vi "WPI_GyroXRS450_SPI_Open.vi"(6 "Calibrated Center Offset":dbl, 7 "Calibration Time (s)":dbl=2.0, 8 "error in":errorcluster, 9 "Calibrate On Open":bool=TRUE, 10 "Sample Rate (Hz)":dbl=2000.0, 11 "SPI Bus":T3) -> (0 "error out":errorcluster, 2 "Calibrated Center Offset Out":dbl, 3 "GyroDevRef":T1={"DevStatus"={"status"=FALSE, "code"=0, "source"=""}, "Analog Channel"=enum."AI 0", "Gain (VoltsPerDegree/Second)"=0.0, "Gyro Type"=enum."Analog", "Handle"=0, "SPI Bus"=enum."Invalid", "Device Found"=FALSE, "Sample Rate"=1.0, "Calibrate On Open"=FALSE, "Offset"=0.0} {"Sample Rate" min=0.25 max=100.0 step=0.25})   [LabVIEW 2017]
doc: "Opens a reference to the gyroscope you specify. You must open a reference before using any other VIs on this palette.\n\nThis software is licensed. Open the labview\\readme\\WPI Robotics Library Open Source License.txt file for more information."
uses:
  <vilib>/Rock Robotics/SystemInterfaces/spilib/spi_bus.ctl
  <vilib>/Rock Robotics/WPI/Gyro/WPI_GyroDevRef.ctl
  <vilib>/Rock Robotics/SystemInterfaces/AI/FPGA_AIChannel.ctl
  <vilib>/Rock Robotics/WPI/SPI/WPI_SPIMode.ctl
  <vilib>/Rock Robotics/WPI/Gyro/ADXRS453/WPI_Gyro_ADXRS453_Commands.ctl
  <vilib>/Rock Robotics/WPI/Gyro/ADXRS453/WPI_Gyro_ADXRS453_Registers.ctl
  <vilib>/Rock Robotics/SystemInterfaces/NetworkCommunication/NetComm_UsageReport_ResourceType.ctl
  <vilib>/Analysis/baseanly.llb/Mean (DBL).vi
  <vilib>/Analysis/NI_AALBase.lvlib
panel:
  # "Analog"
  # "XRS"
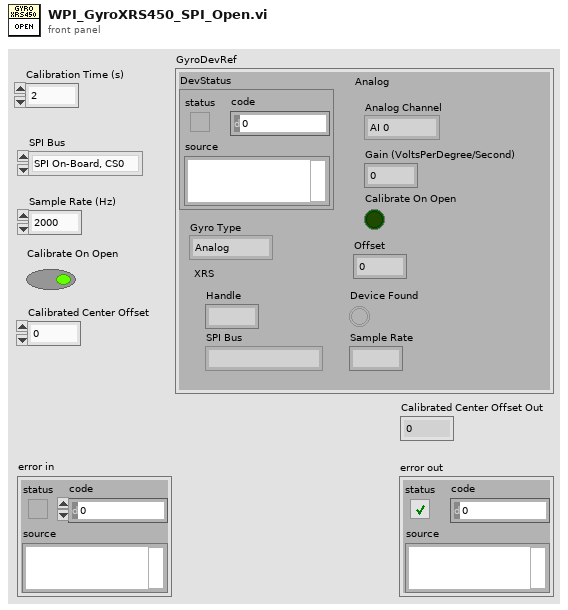
[diagram p1: front panel]
types:
  T1 = typedef "WPI_GyroDevRef.ctl" = cluster{"DevStatus":errorcluster, "Analog Channel":T2, "Gain (VoltsPerDegree/Second)":dbl, "Gyro Type":enum16{"Analog", "XRS450"}, "Handle":i32, "SPI Bus":T3, "Device Found":bool, "Sample Rate":dbl, "Calibrate On Open":bool, "Offset":dbl}
  T2 = typedef "FPGA_AIChannel.ctl" = enum8{"AI 0", "AI 1", "AI 2", "AI 3", "AI MXP 0", "AI MXP 1", "AI MXP 2", "AI MXP 3", "Invalid"}
  T3 = typedef "spi_bus.ctl" = enum16{"SPI On-Board, CS0", "SPI On-Board, CS1", "SPI On-Board, CS2", "SPI On-Board, CS3", "SPI MXP", "Invalid"}
  T4 = typedef "WPI_Gyro_ADXRS453_Commands.ctl" = u8
  T5 = typedef "WPI_SPIMode.ctl" = enum16{"Mode 0 (Clk Idle Low,Sample on Leading)", "Mode 1 (Clk Idle Low,Sample on Trailing)", "Mode 2 (Clk Idle High,Sample on Leading)", "Mode 3 (Clk Idle High,Sample on Trailing)"}
  T6 = typedef "NetComm_UsageReport_ResourceType.ctl" = enum8{"Controller", "Module", "Language", "CANPlugin", "Accelerometer", "ADXL345", "AnalogChannel", "AnalogTrigger", "AnalogTriggerOutput", "CANJaguar", "Compressor", "Counter", "Dashboard", "DigitalInput", "DigitalOutput", "DriverStationCIO", "DriverStationEIO", "DriverStationLCD", "Encoder", "GearTooth", "Gyro", "I2C", "Framework", "Jaguar", "Joystick", "Kinect", "KinectStick", "PIDController", "Preferences", "PWM", "Relay", "RobotDrive", "SerialPort", "Servo", "Solenoid", "SPI", "Task", "Ultrasonic", "Victor", "Button", "Command", "AxisCamera", "PCVideoServer", "SmartDashboard", "Talon", "HiTechnicColorSensor", "HiTechnicAccel", "HiTechnicCompass", "SRF08", "AnalogOutput", "Victor SP", "Talon SRX", "CAN Talon SRX", "ADXL362 Accel", "ADXRS450 Gyro", "Rev SPARK", "Mindsensors SD540", "Digital Filter", "ADIS16448", "PDP", "PCM", "PigeonIMU", "Nidec Brushless", "CTRE CANifier", "CTRE Future 0", "CTRE Future 1", "CTRE Future 2", "CTRE Future 3", "CTRE Future 4", "CTRE Future 5", "CTRE Future 6"}
  T7 = typedef "WPI_Gyro_ADXRS453_Registers.ctl" = u16
  T8 = typedef "WPI_SPIDevRef.ctl" = cluster{"DevStatus":errorcluster, "Handle":i32, "SPI Bus":T3}
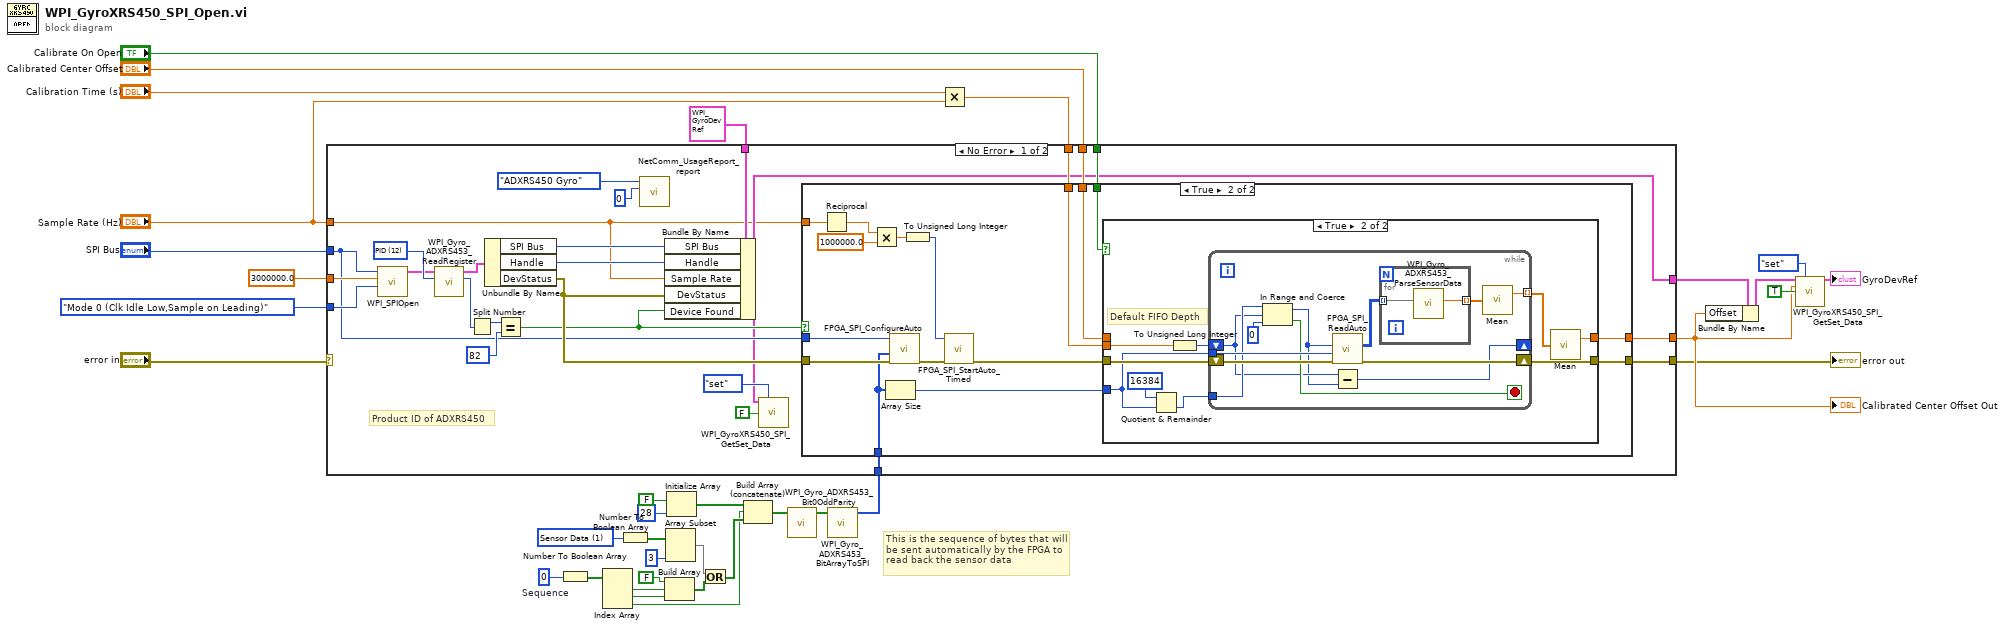
[diagram p0: block diagram]
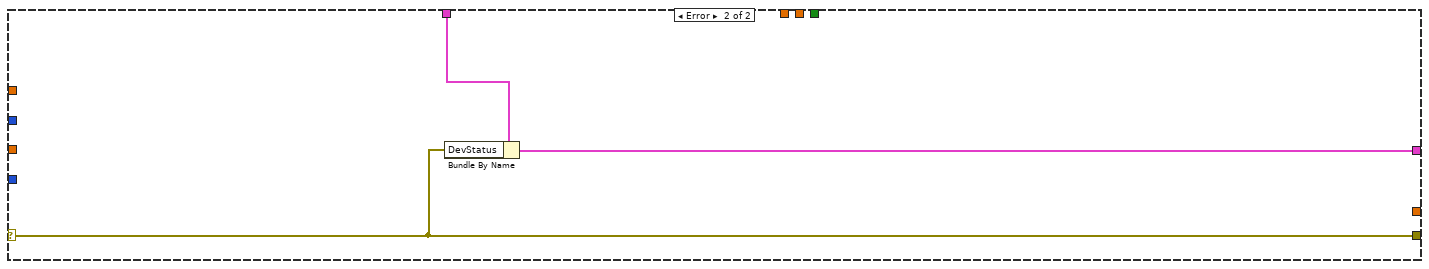
[diagram p4: hidden frame]
diagram:
  w23 = u8 0  # Sequence
  w24 = T4 1 items=["Read"=4, "Write"=2, "Sensor Data"=1]
  # "This is the sequence of bytes that will be sent automatically by the FPGA to read back the sensor data"
  n1 = Number To Boolean Array(number=w23) -> (Boolean array=w22:bool[])
  n2 = Index Array(array=w22) -> (element #1=w21:bool, element #2=w20:bool, element #3=w15:bool)  [unwired: 3 in]
  n3 = Number To Boolean Array(number=w24) -> (Boolean array=w25:bool[])
  n4 = Build Array(FALSE, w21, w20) -> (w18:bool[])
  n5 = Array Subset(array=w25, length=3) -> (w17:bool[])  [unwired: 1 in]
  n6 = Initialize Array(FALSE, 28 ("dimension size")) -> (w30:bool[])
  n7 = Or(x=w17, y=w18) -> (x .or. y?=w16:bool[])
  n8 = Build Array (concatenate)(w30, w15, w16) -> (w29:bool[])
  n9 = call <vilib>:"WPI_Gyro_ADXRS453_Bit0OddParity.vi"("Array in"=w29) -> ("Array out"=w31:bool[])  [unwired: 10 in]
  n10 = call <vilib>:"WPI_Gyro_ADXRS453_BitArrayToSPI.vi"("32-bit Array in"=w31) -> ("SPI Byte Array (MSB first)"=w8:u8[])  [unwired: 10 in]
  n11 = Multiply(x="Calibration Time (s)", y="Sample Rate (Hz)") -> (x*y=w10:dbl)
  n12 = case shown="No Error" "error in" {
    selector: "error in" -> [_ w104]
    tunnel: "SPI Bus" -> [w47 _]
    tunnel: 3000000.0 ("Clock Rate (Hz)") -> [w61 _]
    tunnel: WPI_SPIMode."Mode 0 (Clk Idle Low,Sample on Leading)" ("Mode (3)") -> [w60 _]
    tunnel: T1 {"DevStatus"={"status"=FALSE, "code"=0, "source"=""}, "Analog Channel"=enum."AI 1", "Gain (VoltsPerDegree/Second)"=0.0, "Gyro Type"=enum."XRS450", "Handle"=0, "SPI Bus"=enum."Invalid", "Device Found"=FALSE, "Sample Rate"=1.0, "Calibrate On Open"=FALSE, "Offset"=0.0} ("GyroDeviceRef") -> [w59 w106]
    tunnel: [w37 w105] -> w14
    tunnel: "Sample Rate (Hz)" -> [w36 _]
    tunnel: w8 -> [w43 _]
    tunnel: "Calibrate On Open" -> [w46 _]
    tunnel: w10 -> [w45 _]
    tunnel: "Calibrated Center Offset" -> [w44 _]
    tunnel: [w42 _] -> w4
    tunnel: [w41 w104] -> w3
    frame No Error {
      w55 = T7 12 items=["Rate"=0, "Tem"=2, "LoCST"=4, "HiCST"=6, "Quad"=8, "Fault"=10, "PID"=12, "SN High"=14, "SN Low"=16]
      # "Product ID of ADXRS450"
      n13 = call <vilib>:"WPI_SPIOpen.vi"("Mode (3)"=w60, "Clock Rate (Hz)"=w61, "SPI Bus"=w47) -> ("SPIDevRef"=w51:T8)  [unwired: 7 in, 1 out]
      n14 = call <vilib>:"WPI_Gyro_ADXRS453_ReadRegister.vi"("ADXRS453 Register"=w55, "SPIDevRef in"=w51) -> ("Register Value"=w54:u16, "SPIDevRef out"=w50:T8)  [unwired: 7 in, 1 out]
      n15 = Split Number(x=w54) -> (hi(x)=w53:u8)  [unwired: 1 out]
      n16 = Unbundle By Name(w50) -> ("SPI Bus"=w58:T3, "Handle"=w57:i32, "DevStatus"=w56:errorcluster)
      n17 = Equal?(x=w53, y=u8 82) -> (x = y?=w40:bool)
      n18 = call <vilib>:"NetComm_UsageReport_report.vi"("Instance Number"=u8 0, "Resource Type"=NetComm_UsageReport_ResourceType."ADXRS450 Gyro") -> ()  [unwired: 10 in]
      n19 = Bundle By Name(cluster=w59, "SPI Bus"=w58, "Handle"=w57, "Sample Rate"=w36, "DevStatus"=w56, "Device Found"=w40) -> (w37:T1)
      n20 = call <vilib>:"WPI_GyroXRS450_SPI_GetSet_Data.vi"("GyroDeviceRef"=w37, "Operation"=enum16{"set", "get"}."set", "Calibrated"=FALSE) -> ()  [unwired: 8 in, 5 out]
      n21 = case shown="True" w40 {
        tunnel: w56 -> [w62 w78]
        tunnel: w47 -> [_ w77]
        tunnel: w36 -> [_ w72]
        tunnel: w46 -> [_ w70]
        tunnel: w45 -> [_ w69]
        tunnel: w44 -> [_ w68]
        tunnel: w43 -> [_ w66]
        tunnel: [_ w65] -> w42
        tunnel: [w62 w64] -> w41
        frame False {
        }
        frame True {
          n22 = Reciprocal(x=w72) -> (1/x=w63:dbl)
          n23 = Multiply(x=w63, y=1000000.0 ("x")) -> (x*y=w75:dbl)
          n24 = Array Size(array=w66) -> (size(s)=w71:i32)
          n25 = call <vilib>:"FPGA_SPI_ConfigureAuto.vi"("error in"=w78, "SPI Auto TX Byte Array"=w66, "SPI Bus"=w77) -> ("error out"=w74:errorcluster)  [unwired: 8 in]
          n26 = To Unsigned Long Integer(number=w75) -> (unsigned 32bit integer=w76:u32)
          n27 = call <vilib>:"FPGA_SPI_StartAuto_Timed.vi"("error in (no error)"=w74, "Sample Period (us)"=w76) -> ("error out"=w67:errorcluster)  [unwired: 9 in]
          n28 = case shown="True" w70 {
            tunnel: w69 -> [_ w89]
            tunnel: w68 -> [w80 _]
            tunnel: [w80 w82] -> w65
            tunnel: w67 -> [w79 w88]
            tunnel: w71 -> [_ w83]
            tunnel: [w79 w86] -> w64
            frame False {
            }
            frame True {
              # "Default FIFO Depth"
              n29 = Quotient & Remainder(x=u32 16384 ("unsigned 32bit integer"), y=w83) -> (floor(x/y)=w81:u32)  [unwired: 1 out]
              n30 = To Unsigned Long Integer(number=w89) -> (unsigned 32bit integer=w87:u32)
              n31 = while {
                tunnel: [w97] -> w85 mode=indexing
                tunnel: w83 -> [w96]
                shift-right: [w98] -> w86
                shift-left: w88 -> [w100]
                tunnel: w81 -> [w95]
                shift-right: [w90] -> _
                shift-left: w87 -> [w92]
                stop <- w93 stop-if-true
                n32 = In Range and Coerce(upper limit=w95, x=w92, lower limit=u32 0) -> (coerced(x)=w91:u32, In Range?=w93:bool)
                n33 = call <vilib>:"FPGA_SPI_ReadAuto.vi"("error in (no error)"=w100, "Bytes per Sample"=w96, "Samples to Read"=w91) -> ("error out"=w98:errorcluster, "Data"=w99:u8[][])  [unwired: 7 in]
                n34 = Subtract(x=w92, y=w91) -> (x-y=w90:u32)
                n35 = for {
                  tunnel: w99 -> [w103] mode=indexing
                  tunnel: [w102] -> w101 mode=indexing
                  # "Offset Calibration"
                  n36 = call <vilib>:"WPI_Gyro_ADXRS453_ParseSensorData.vi"("Data"=w103) -> ("Angular Rate (deg/sec)"=w102:dbl)  [unwired: 8 in, 2 out]
                }
                n37 = call-poly <vilib>:"Mean.vi"("X"=w101) -> ("mean"=w97:dbl)  [unwired: 1 out]
              }
              n38 = call-poly <vilib>:"Mean.vi"("X"=w85) -> ("mean"=w82:dbl)  [unwired: 1 out]
            }
          }
        }
      }
    }
    frame Error {
      n39 = Bundle By Name(cluster=w106, "DevStatus"=w104) -> (w105:T1)
    }
  }
  "error out" <- w3
  "Calibrated Center Offset Out" <- w4
  n40 = Bundle By Name(cluster=w14, "Offset"=w4) -> (w2:T1)
  n41 = call <vilib>:"WPI_GyroXRS450_SPI_GetSet_Data.vi"("GyroDeviceRef"=w2, "Operation"=enum16{"set", "get"}."set", "Offset"=w4, "Calibrated"=TRUE) -> ("GyroDeviceRef"=→"GyroDevRef":T1)  [unwired: 7 in, 4 out]
